vi "GetJoystickValues.vi"(0 "JoystickDevRef":T1) -> (1 "Axes":dbl[](array[numeric]), 2 "Buttons":bool[](array[boolean]))   [LabVIEW 2015]
uses:
  <vilib>/Rock Robotics/WPI/Joystick/WPI_JoystickDevRef.ctl
  <vilib>/Rock Robotics/WPI/Joystick/WPI_JoystickDeviceEnum.ctl
  <vilib>/Rock Robotics/WPI/DriverStation/WPI_DriverStationRobotMode2.ctl
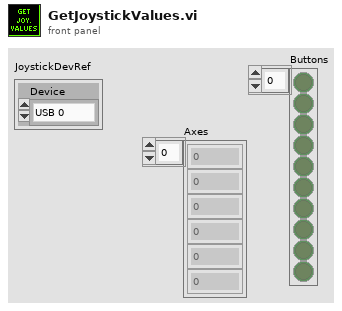
[diagram p1: front panel]
types:
  T1 = typedef "WPI_JoystickDevRef.ctl" = cluster{"Device":T2}
  T2 = typedef "WPI_JoystickDeviceEnum.ctl" = enum16{"USB 0", "USB 1", "USB 2", "USB 3", "USB 4", "USB 5"}
  T3 = typedef "WPI_DriverStationRobotMode2.ctl" = enum16{"Autonomous Disabled", "Autonomous Enabled", "Teleop Disabled", "Teleop Enabled", "Disconnected", "Finish", "Test Disabled", "Test Enabled", "Emergency Stopped"}
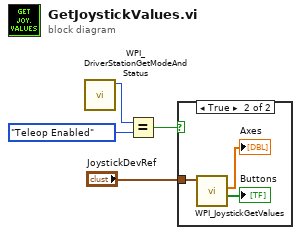
[diagram p0: block diagram]
diagram:
  n1 = call <vilib>:"WPI_DriverStationGetModeAndStatus.vi"() -> ("Robot Mode"=w3:T3)  [unwired: 10 in, 1 out]
  n2 = Equal?(x=w3, y=WPI_DriverStationRobotMode2."Teleop Enabled") -> (x = y?=w1:bool)
  n3 = case shown="True" w1 {
    tunnel: "JoystickDevRef" -> [_ w7]
    frame False {
    }
    frame True {
      n4 = call <vilib>:"WPI_JoystickGetValues.vi"("JoystickDevRef"=w7) -> ("Buttons"=→"Buttons":bool[], "Axes"=→"Axes":dbl[])  [unwired: 6 in, 3 out]
    }
  }
